vi "write char.vi"(8 "error in (no error)":errorcluster, 10 "write buffer":string, 11 "Serial port":refnum<visa-resource-name>) -> (0 "error out":errorcluster, 2 "read buffer":string, 3 "Serial Port":refnum<visa-resource-name>)   [LabVIEW 2010]
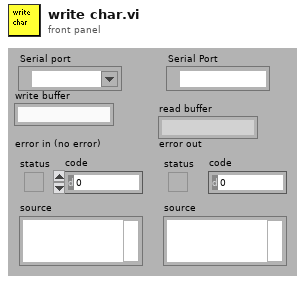
[diagram p1: front panel]
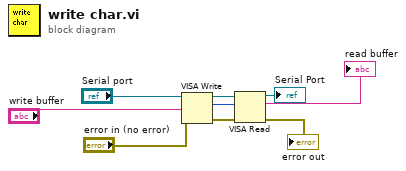
[diagram p0: block diagram]
diagram:
  n1 = VISA Write(VISA resource name="Serial port", write buffer="write buffer", error in (no error)="error in (no error)") -> (VISA resource name out=w9:refnum<visa-resource-name>, return count=w8:u32, error out=w7:errorcluster)
  n2 = VISA Read(VISA resource name=w9, byte count=w8, error in (no error)=w7) -> (VISA resource name out=→"Serial Port":refnum<visa-resource-name>, read buffer=→"read buffer":string, error out=→"error out":errorcluster)  [unwired: 1 out]
